vi "StringToDateTime.vi"(10 "error in (no error)":errorcluster, 11 "datetime string":string) -> (2 "error out":errorcluster, 3 "timestamp":timestamp)   [LabVIEW 2019, in "ByteQXWebAPI.lvlib" / "ByteQXAPIBase.lvclass"]
doc: "Cast a String date into a Labview date"
uses:
  ByteQXAPIBase.lvclass
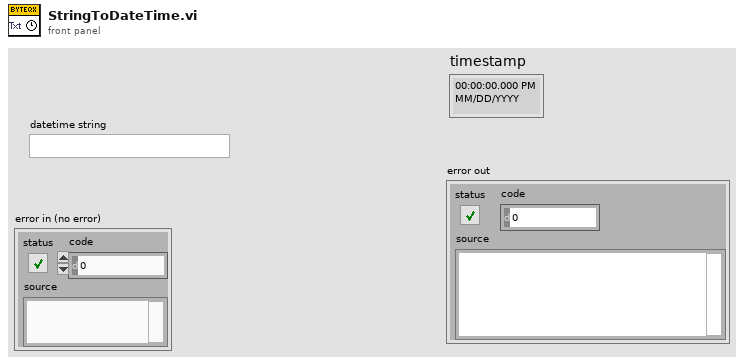
[diagram p1: front panel]
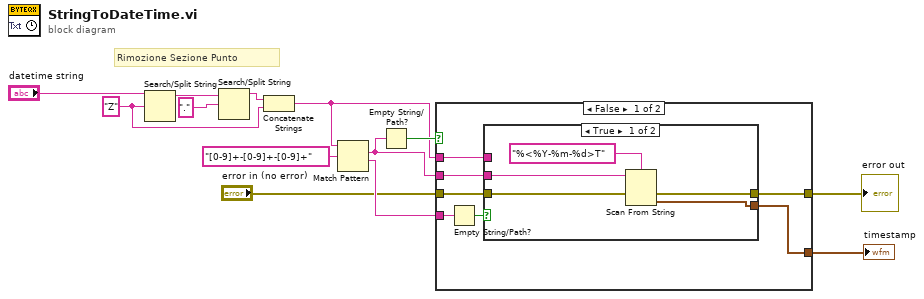
[diagram p0: block diagram]
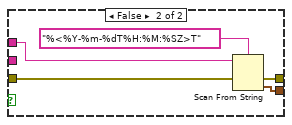
[diagram p2: hidden frame]
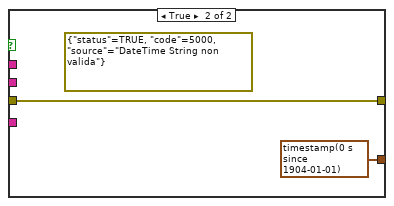
[diagram p3: hidden frame]
diagram:
  w5 = "Z" ("search string/char (-)")
  # "Rimozione Sezione Punto"
  n1 = Search/Split String(string="datetime string", search string/char (-)=w5) -> (substring before match=w8:string)  [unwired: 1 in, 2 out]
  n2 = Search/Split String(string=w8, search string/char (-)=".") -> (substring before match=w6:string)  [unwired: 1 in, 2 out]
  n3 = Concatenate Strings(w6, w5) -> (w4:string)
  n4 = Match Pattern(string=w4, regular expression="[0-9]+-[0-9]+-[0-9]+") -> (match substring=w10:string, after substring=w11:string)  [unwired: 1 in, 2 out]
  n5 = Empty String/Path?(string/path=w10) -> (empty?=w12:bool)
  n6 = case shown="False" w12 {
    tunnel: [w19 timestamp(0 s since 1904-01-01)] -> w1
    tunnel: w10 -> [w20 _]
    tunnel: w11 -> [w17 _]
    tunnel: w4 -> [w16 _]
    tunnel: "error in (no error)" -> [w15 w31]
    tunnel: [w14 w31] -> w2
    frame False {
      n7 = Empty String/Path?(string/path=w17) -> (empty?=w18:bool)
      n8 = case shown="True" w18 {
        tunnel: w20 -> [w25 _]
        tunnel: [w24 w30] -> w19
        tunnel: w16 -> [_ w28]
        tunnel: w15 -> [w22 w26]
        tunnel: [w21 w27] -> w14
        frame True {
          n9 = Scan From String(format string="%<%Y-%m-%d>T", input string=w25, error in=w22) -> (error out=w21:errorcluster, output 1=w24:timestamp)  [unwired: 2 in, 2 out]
        }
        frame False {
          n10 = Scan From String(format string="%<%Y-%m-%dT%H:%M:%SZ>T", input string=w28, error in=w26) -> (error out=w27:errorcluster, output 1=w30:timestamp)  [unwired: 2 in, 2 out]
        }
      }
    }
    frame True {
      (unwired) errorcluster {"status"=TRUE, "code"=5000, "source"="DateTime String non valida"} ("error IO")
    }
  }
  "timestamp" <- w1
  "error out" <- w2
